vi "Example of Basic Features.vi"   [LabVIEW 2016]
uses:
  <userlib>/_MGI/User Interface/Progress Bar/Progress Bar.lvclass
panel:
  # "Run this VI and watch the show on the LabVIEW Taskbar button!"
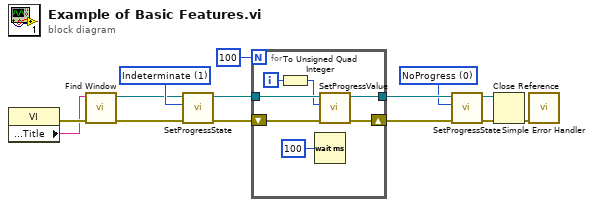
[diagram p0: block diagram]
diagram:
  w2 = 0 items=["NoProgress"=0, "Indeterminate"=1, "Normal"=2, "Error"=4, "Paused"=8] ("State (No Progress)")
  w10 = 1 items=["NoProgress"=0, "Indeterminate"=1, "Normal"=2, "Error"=4, "Paused"=8] ("state")
  n1 = property class="VI"() -> (error out=w13:errorcluster, "Front Panel.Title"=w12:string)  [unwired: 2 in, 1 out]
  n2 = call <userlib>:"Find Window.vi"("error in (no error)"=w13, "Window Title (Callers Window)"=w12) -> ("error out"=w11:errorcluster, "Window Handle"=w9:refnum<k24>)  [unwired: 8 in]
  n3 = call <userlib>:"SetProgressState.vi"("error in (no error)"=w11, "State (No Progress)"=w10, "Window Handle"=w9) -> ("error out"=w8:errorcluster, "dup Window Handle"=w7:refnum<k24>)  [unwired: 7 in]
  n4 = for {
    N: 100 -> [_]
    tunnel: w7 -> [w20]
    shift-right: [w17] -> w4
    shift-left: w8 -> [w21]
    tunnel: [w15] -> w5
    i -> [w19]
    n5 = To Unsigned Quad Integer(1:w19) -> (0:w18:u64)
    n6 = Wait (ms)(milliseconds to wait=u32 100) -> ()  [unwired: 1 out]
    n7 = call <userlib>:"SetProgressValue.vi"("error in (no error)"=w21, "current (0)"=w18, "Window Handle"=w20) -> ("error out"=w17:errorcluster, "dup Window Handle"=w15:refnum<k24>)  [unwired: 7 in]
  }
  n8 = call <userlib>:"SetProgressState.vi"("error in (no error)"=w4, "State (No Progress)"=w2, "Window Handle"=w5) -> ("error out"=w3:errorcluster, "dup Window Handle"=w1:refnum<k24>)  [unwired: 7 in]
  n9 = Close Reference(reference=w1, error in (no error)=w3) -> (error out=w14:errorcluster)
  n10 = call <vilib>:"Simple Error Handler.vi"("error in (no error)"=w14) -> ()  [unwired: 4 in, 5 out]
